vi "Normal.vi"(0 "class data in":refnum<class "LvNative.lvclass">, 5 "error in (no error)":errorcluster) -> (14 "class data out":refnum<class "LvNative.lvclass">, 19 "error out":errorcluster)   [LabVIEW 2020, in "G#MethodTemplates.lvclass"]
uses:
  <vilib>/addons/_AddQ/G#Templates/G#MethodTemplates/G#MethodTemplates.lvclass
  <vilib>/addons/_AddQ/G#Templates/LvNative/LvNative.lvclass
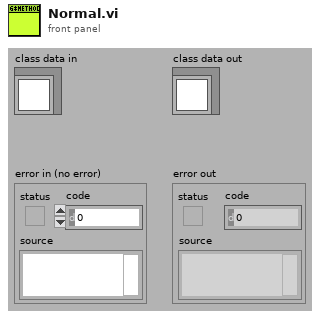
[diagram p1: front panel]
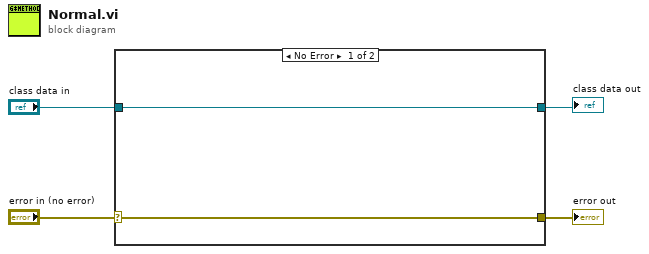
[diagram p0: block diagram]
diagram:
  n1 = case shown="No Error" "error in (no error)" {
    selector: "error in (no error)" -> [w6 w8]
    tunnel: [w6 w8] -> w3
    tunnel: "class data in" -> [w5 w7]
    tunnel: [w5 w7] -> w1
    frame No Error {
    }
    frame Error {
    }
  }
  "error out" <- w3
  "class data out" <- w1
